vi "GetUSAFACTS.vi"(11 "index":enum16{"Confirmed", "Deaths", "Population"}(ring)) -> (2 "Data":string[][](array[string]), 3 "body":string)   [LabVIEW 2017]
uses:
  <vilib>/httpClient/LabVIEWHTTPClient.lvlib
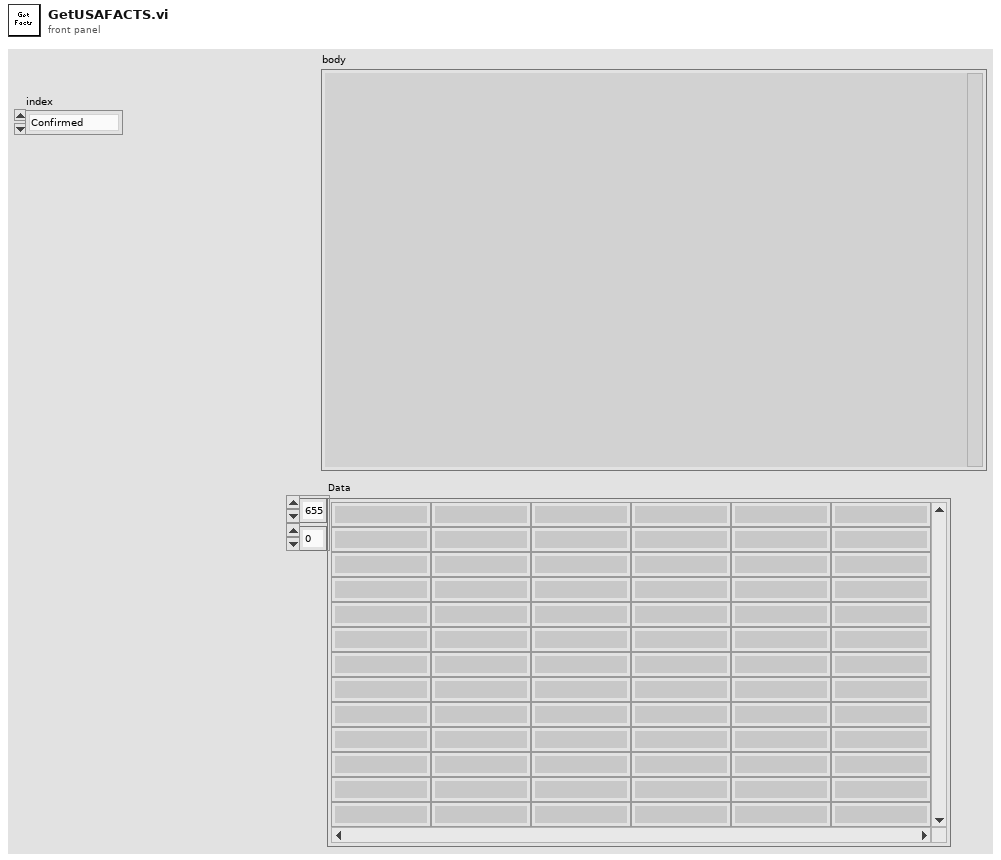
[diagram p1: front panel]
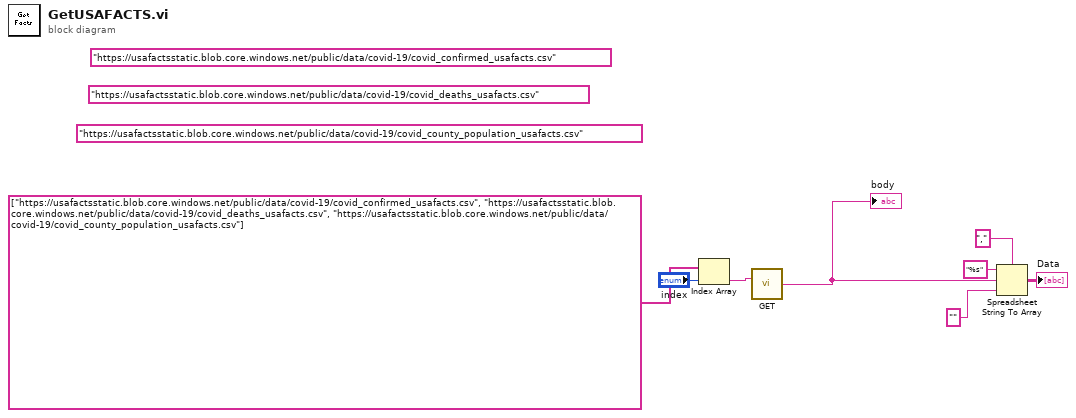
[diagram p0: block diagram]
diagram:
  (unwired) "https://usafactsstatic.blob.core.windows.net/public/data/covid-19/covid_county_population_usafacts.csv" ("url")
  (unwired) "https://usafactsstatic.blob.core.windows.net/public/data/covid-19/covid_deaths_usafacts.csv" ("url")
  (unwired) "https://usafactsstatic.blob.core.windows.net/public/data/covid-19/covid_confirmed_usafacts.csv" ("url")
  n1 = Index Array(array=string[] ["https://usafactsstatic.blob.core.windows.net/public/data/covid-19/covid_confirmed_usafacts.csv", "https://usafactsstatic.blob.core.windows.net/public/data/covid-19/covid_deaths_usafacts.csv", "https://usafactsstatic.blob.core.windows.net/public/data/covid-19/covid_county_population_usafacts.csv"], index="index") -> (element=w2:string)
  n2 = call <vilib>:"GET.vi"("url"=w2) -> ("body"=w8:string)  [unwired: 11 in, 3 out]
  "body" <- w8
  n3 = Spreadsheet String To Array(delimiter (Tab)=",", format string="%s", spreadsheet string=w8, array type (2D Dbl)="") -> (array=→"Data":string[][])
